vi "Config.Read UUT Info.vi"(8 "error in (no error)":errorcluster, 9 "Default Process Step":string="Undefined", 10 "Default Product Name":string="Undefined", 11 "Local Station Config File":path) -> (0 "error out":errorcluster, 2 "Process Step":string, 3 "Product":string)   [LabVIEW 2018]
uses:
  <vilib>/Utility/config.llb/Read Key (String).vi
  <vilib>/Utility/config.llb/NI_LVConfig.lvlib
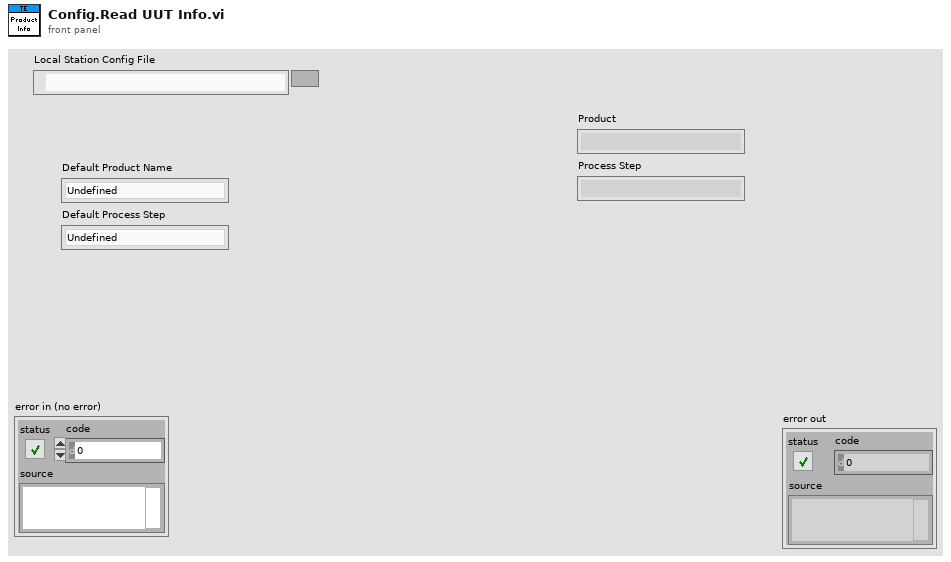
[diagram p1: front panel]
types:
  T1 = typedef "NI_LVConfig.lvlib/Config Data RefNum.ctl" = refnum<k1>
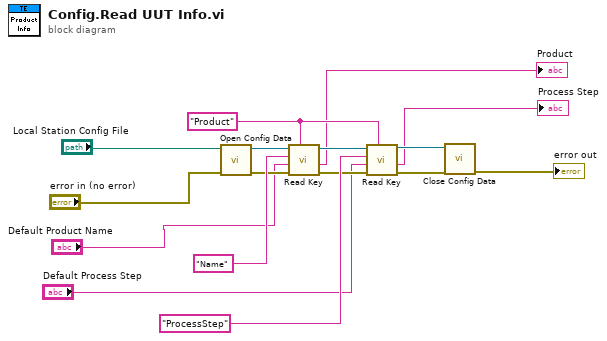
[diagram p0: block diagram]
diagram:
  w10 = "Product"
  n1 = call <vilib>:"Open Config Data.vi"("error in (no error)"="error in (no error)", "configuration file path"="Local Station Config File") -> ("error out"=w11:errorcluster, "refnum"=w13:T1)  [unwired: 7 in, 1 out]
  n2 = call-poly <vilib>:"Read Key.vi"("section"=w10, "error in (no error)"=w11, "default value"="Default Product Name", "key"="Name", "refnum"=w13) -> ("error out"=w12:errorcluster, "value"=→"Product":string, "refnum out"=w14:T1)  [unwired: 3 in, 1 out]
  n3 = call-poly <vilib>:"Read Key.vi"("section"=w10, "error in (no error)"=w12, "default value"="Default Process Step", "key"="ProcessStep", "refnum"=w14) -> ("error out"=w5:errorcluster, "value"=→"Process Step":string, "refnum out"=w6:T1)  [unwired: 3 in, 1 out]
  n4 = call <vilib>:"Close Config Data.vi"("error in (no error)"=w5, "refnum"=w6) -> ("error out"=→"error out":errorcluster)  [unwired: 8 in, 1 out]
